vi "mkSetMode.vi"(9 "Camera in":T1={"Frame rate (Hz)"=10, "Gain [1-4]"=1024.0, "Offset"=75, "Exposure time"=50, "Mode"=1000, "ROIs"=[], "ROI Size"={"X"=0, "Y"=0}, "Number of buffers"=40} {"Exposure time" min=50}, 11 "IMAQ Refnum in":refnum<k11>) -> (1 "Camera Settings":T1={"Frame rate (Hz)"=10, "Gain [1-4]"=1024.0, "Offset"=75, "Exposure time"=50, "Mode"=1000, "ROIs"=[], "ROI Size"={"X"=0, "Y"=0}, "Number of buffers"=40} {"Exposure time" min=50}, 2 "Camera Mode [out]":i32, 3 "IMAQ Refnum out":refnum<k11>)   [LabVIEW 2011]
uses:
  CameraConfig.ctl
panel:
  out "String Read":string
  # "us"
  # "us"
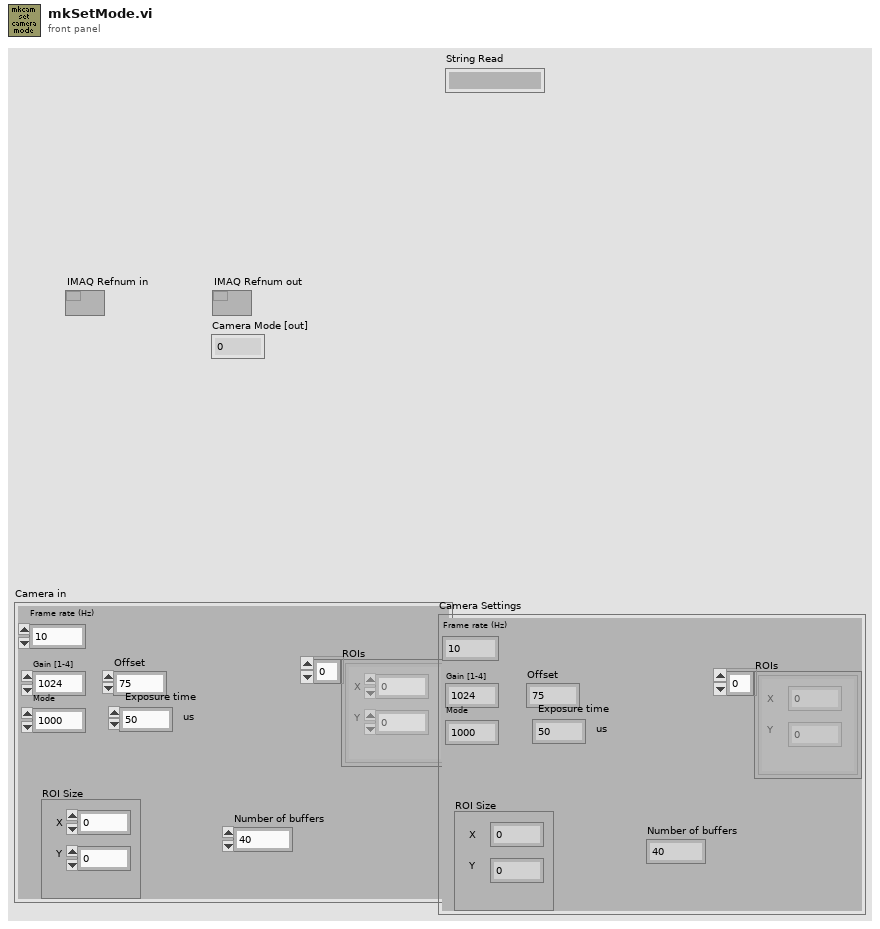
[diagram p1: front panel]
types:
  T1 = typedef "CameraConfig.ctl" = cluster{"Frame rate (Hz)":u32, "Gain [1-4]":sgl, "Offset":i16, "Exposure time":i32, "Mode":i16, "ROIs":cluster{"X":i32, "Y":i32}[], "ROI Size":cluster{"X":i32, "Y":i32}, "Number of buffers":i32}
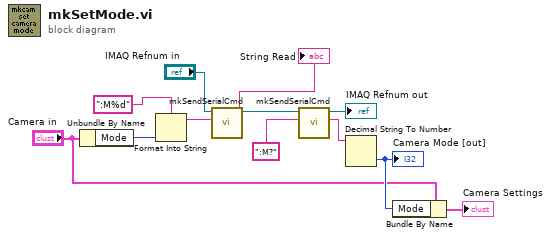
[diagram p0: block diagram]
diagram:
  n1 = Unbundle By Name("Camera in") -> ("Mode"=w2:i16)
  n2 = Format Into String(format string=":M%d", w2) -> (resulting string=w10:string)  [unwired: 2 in, 1 out]
  n3 = call "mkSendSerialCmd.vi"("String"=w10, "IMAQ Refnum in"="IMAQ Refnum in") -> ("String Read"=→"String Read":string, "IMAQ Refnum out"=w8:refnum<k11>)  [unwired: 6 in, 2 out]
  n4 = call "mkSendSerialCmd.vi"("String"=":M?", "IMAQ Refnum in"=w8) -> ("String Read"=w6:string, "IMAQ Refnum out"=→"IMAQ Refnum out":refnum<k11>)  [unwired: 6 in, 2 out]
  n5 = Decimal String To Number(string=w6) -> (number=w5:i32)  [unwired: 2 in, 1 out]
  "Camera Mode [out]" <- w5
  n6 = Bundle By Name(cluster="Camera in", "Mode"=w5) -> (→"Camera Settings":T1)
